vi "AdaptToInputs.vi"(3 "Term Types":T1[](array[typedef]), 4 "XRef":refnum<vi>, 5 "State In":T4={"Output Type"=variant(dbl 0.0), "Typedef Name"="", "Input Type"=variant, "Constant Types"=[], "Error"={"status"=FALSE, "code"=0, "source"=""}, "Typedef Path"=path "", "Names"=[], "Event Cluster Name"=""}) -> (0 "Reply":string[](array[string]), 2 "State Out":T4={"Output Type"=variant(dbl 0.0), "Typedef Name"="", "Input Type"=variant, "Constant Types"=[], "Error"={"status"=FALSE, "code"=0, "source"=""}, "Typedef Path"=path "", "Names"=[], "Event Cluster Name"=""})   [LabVIEW 2015, in "Create-Signals.xnode"]
doc: "This ability VI is called by LabVIEW during type propagation so that your XNode may adapt itself to new input types. Term Types is an array of pairs of current Term IDs and the type descriptors corresponding to them. The type descriptors are taken from the signal connected to the terminal. Unwired terminals are not included in the array. Use Reply to inform LabVIEW of any actions it needs to take.\n\nDefault behavior: None.\n\nThis ability does not provide UI and OS messages are not handled."
uses:
  Create-Signals.xnode
  State.ctl
  <vilib>/XNodeSupport/XNodeTermTypeIDPair.ctl
  <vilib>/XNodeSupport/XNodeType.ctl
  <vilib>/XNodeSupport/XNodeString.ctl
  <vilib>/Utility/Data Type/Type Definitions/Refnum Type.ctl
  <vilib>/LV-Scripting/LV-Scripting.lvlib
  <vilib>/Utility/Data Type/NI_Data Type.lvlib
  <vilib>/XNodeSupport/NI_XNodeSupport.lvlib
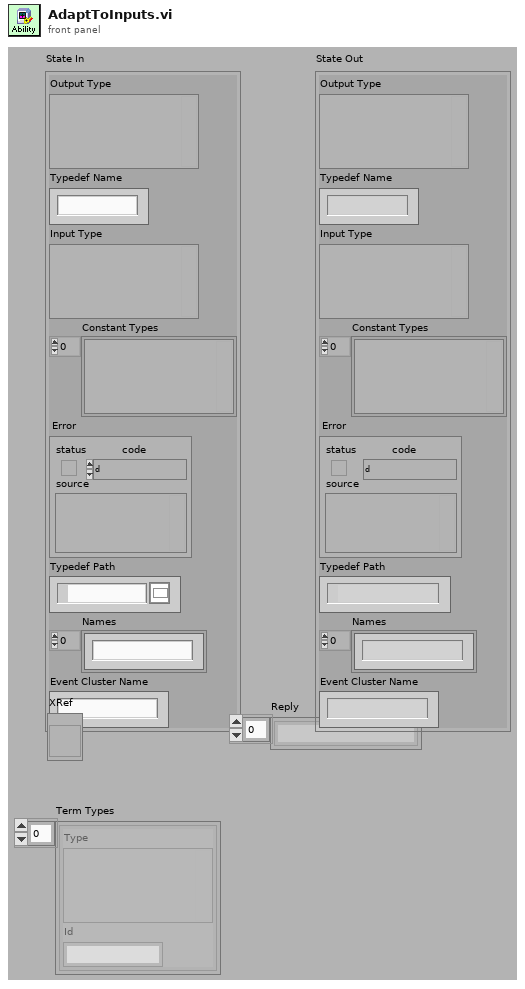
[diagram p1: front panel]
types:
  T1 = typedef "NI_XNodeSupport.lvlib/XNodeTermTypeIDPair.ctl" = cluster{"Type":T2, "Id":T3}
  T2 = typedef "NI_XNodeSupport.lvlib/XNodeType.ctl" = variant
  T3 = typedef "NI_XNodeSupport.lvlib/XNodeString.ctl" = string
  T4 = typedef "Create-Signals.xnode/State.ctl" = cluster{"Output Type":variant, "Typedef Name":string, "Input Type":variant, "Constant Types":variant[], "Error":errorcluster, "Typedef Path":path, "Names":string[], "Event Cluster Name":string}
  T5 = typedef "NI_Data Type.lvlib/Refnum Type.ctl" = enum16{"NotARefnum", "UnknownRefnum", "Generic", "Datalog", "ByteStream", "Device", "Occurence", "TCPNetConnection", "Auto", "Menu", "Imaq", "Hardware", "DataSocket", "Visa", "IVI", "UDPNetConnection", "Notifier", "Queue", "Irda", "EventReg", "DotNet", "UserEvent", "Callback", "UNUSED_EMPTY_POSITION", "BlueToothNetConnection", "LVObjApp", "LVObjVI", "LVObjUnknown", "GenericClass", "UserDefinedRefnumTag", "DataValue", "RT FIFO", "TDMS File"}
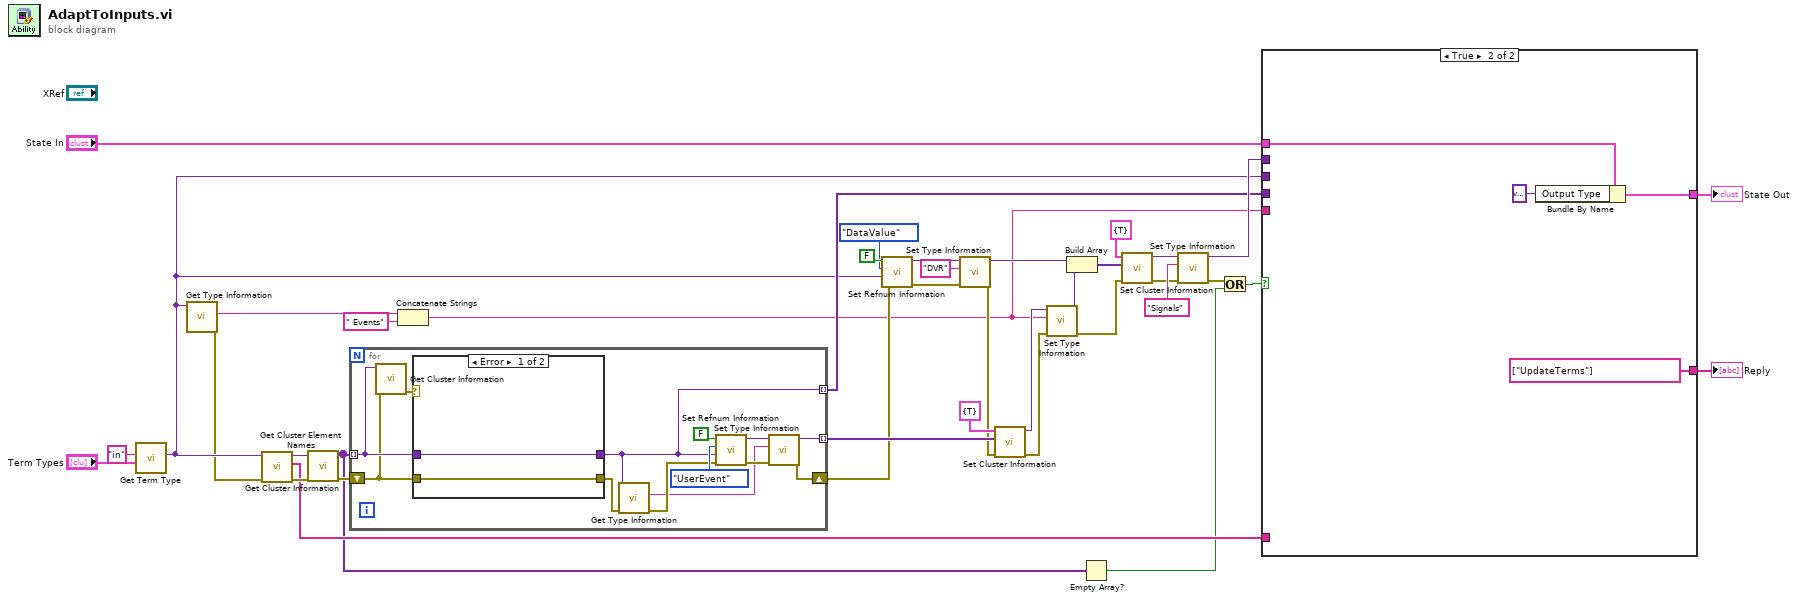
[diagram p0: block diagram]
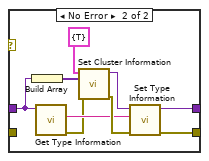
[diagram p2: hidden frame]
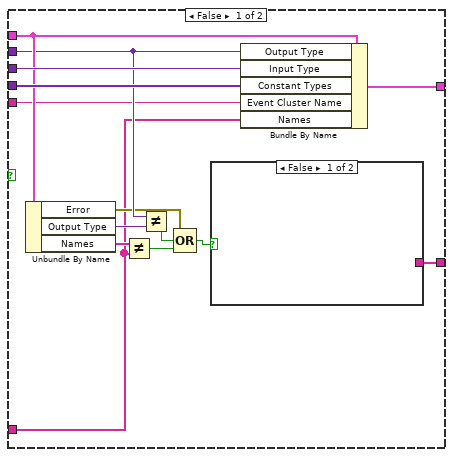
[diagram p3: hidden frame]
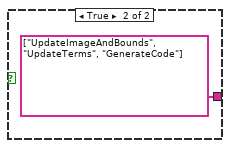
[diagram p4: hidden frame]
diagram:
  n1 = call <vilib>:"Get Term Type.vi"("Term Types"="Term Types", "ID"="in") -> ("Type"=w6:variant)  [unwired: 9 in]
  n2 = call <vilib>:"Get Type Information.vi"("Variant"=w6) -> ("error out"=w5:errorcluster, "Name"=w14:string)  [unwired: 6 in, 3 out]
  n3 = call <vilib>:"Get Cluster Element Names.vi"("error in (no error)"=w5, "Cluster in"=w6) -> ("error out"=w8:errorcluster, "Names"=w4:string[], "Cluster  out"=w7:variant)  [unwired: 7 in]
  n4 = call <vilib>:"Get Cluster Information.vi"("error in (no error)"=w8, "Variant"=w7) -> ("error out"=w24:errorcluster, "Cluster Elements"=w2:variant[])  [unwired: 8 in]
  n5 = for {
    shift-right: [w45] -> w23
    shift-left: w24 -> [w44]
    tunnel: w2 -> [w51] mode=indexing
    tunnel: [w47] -> w36 mode=indexing
    tunnel: [w42] -> w15 mode=indexing
    n6 = call <vilib>:"Get Cluster Information.vi"("error in (no error)"=w44, "Variant"=w51) -> ("error out"=w52:errorcluster)  [unwired: 8 in, 1 out]
    n7 = case shown="Error" w52 {
      tunnel: [w54 w61] -> w42
      tunnel: w51 -> [w54 w57]
      tunnel: [w53 w58] -> w43
      tunnel: w44 -> [w53 _]
      frame Error {
      }
      frame No Error {
        n8 = Build Array(w57) -> (w63:variant[])
        n9 = call <vilib>:"Get Type Information.vi"("Variant"=w57) -> ("error out"=w55:errorcluster, "Name"=w56:string)  [unwired: 6 in, 3 out]
        n10 = call <vilib>:"Set Cluster Information.vi"("error in (no error)"=w55, "Cluster Elements"=w63, "Variant in"=cluster{bool} {TRUE}) -> ("error out"=w59:errorcluster, "Variant out"=w62:variant)  [unwired: 7 in]
        n11 = call <vilib>:"Set Type Information.vi"("error in (no error)"=w59, "Name"=w56, "Variant in"=w62) -> ("error out"=w58:errorcluster, "Variant out"=w61:variant)  [unwired: 7 in]
      }
    }
    n12 = call <vilib>:"Get Type Information.vi"("error in (no error)"=w43, "Variant"=w42) -> ("error out"=w41:errorcluster, "Name"=w40:string)  [unwired: 5 in, 3 out]
    n13 = call <vilib>:"Set Refnum Information.vi"("error in (no error)"=w41, "Strict Type"=w42, "Reference Type"=Refnum_Type."UserEvent", "Variant in"=FALSE) -> ("error out"=w46:errorcluster, "Variant out"=w48:variant)  [unwired: 6 in]
    n14 = call <vilib>:"Set Type Information.vi"("error in (no error)"=w46, "Name"=w40, "Variant in"=w48) -> ("error out"=w45:errorcluster, "Variant out"=w47:variant)  [unwired: 7 in]
  }
  n15 = Concatenate Strings(w14, " Events" ("string")) -> (w9:string)
  n16 = call <vilib>:"Set Refnum Information.vi"("error in (no error)"=w23, "Strict Type"=w6, "Reference Type"=Refnum_Type."DataValue", "Variant in"=FALSE) -> ("error out"=w22:errorcluster, "Variant out"=w33:variant)  [unwired: 6 in]
  n17 = call <vilib>:"Set Type Information.vi"("error in (no error)"=w22, "Name"="DVR", "Variant in"=w33) -> ("error out"=w21:errorcluster, "Variant out"=w30:variant)  [unwired: 7 in]
  n18 = call <vilib>:"Set Cluster Information.vi"("error in (no error)"=w21, "Cluster Elements"=w36, "Variant in"=cluster{bool} {TRUE}) -> ("error out"=w20:errorcluster, "Variant out"=w31:variant)  [unwired: 7 in]
  n19 = call <vilib>:"Set Type Information.vi"("error in (no error)"=w20, "Name"=w9, "Variant in"=w31) -> ("error out"=w19:errorcluster, "Variant out"=w29:variant)  [unwired: 7 in]
  n20 = Build Array(w30, w29) -> (w27:variant[])
  n21 = Empty Array?(array=w2) -> (empty?=w1:bool)
  n22 = call <vilib>:"Set Cluster Information.vi"("error in (no error)"=w19, "Cluster Elements"=w27, "Variant in"=cluster{bool} {TRUE}) -> ("error out"=w18:errorcluster, "Variant out"=w26:variant)  [unwired: 7 in]
  n23 = call <vilib>:"Set Type Information.vi"("error in (no error)"=w18, "Name"="Signals", "Variant in"=w26) -> ("error out"=w17:errorcluster, "Variant out"=w16:variant)  [unwired: 7 in]
  n24 = Or(x=w17, y=w1) -> (x .or. y?=w3:bool)
  n25 = case shown="True" w3 {
    tunnel: [w77 string[] ["UpdateTerms"] ("Reply")] -> w11
    tunnel: "State In" -> [w73 w81]
    tunnel: [w76 w80] -> w10
    tunnel: w16 -> [w71 _]
    tunnel: w6 -> [w75 _]
    tunnel: w15 -> [w74 _]
    tunnel: w9 -> [w66 _]
    tunnel: w4 -> [w64 _]
    frame False {
      n26 = Unbundle By Name(w73) -> ("Error"=w65:errorcluster, "Output Type"=w72:variant, "Names"=w70:string[])
      n27 = Not Equal?(x=w70, y=w64) -> (x != y?=w69:bool)
      n28 = Not Equal?(x=w71, y=w72) -> (x != y?=w68:bool)
      n29 = Compound Arithmetic op=OR(w65, w68, w69) -> (w67:bool)
      n30 = case shown="False" w67 {
        tunnel: [_ string[] ["UpdateImageAndBounds", "UpdateTerms", "GenerateCode"] ("Reply")] -> w77
        frame False {
        }
        frame True {
        }
      }
      n31 = Bundle By Name(cluster=w73, "Output Type"=w71, "Input Type"=w75, "Constant Types"=w74, "Event Cluster Name"=w66, "Names"=w64) -> (w76:T4)
    }
    frame True {
      n32 = Bundle By Name(cluster=w81, "Output Type"=variant) -> (w80:T4)
    }
  }
  "Reply" <- w11
  "State Out" <- w10
